vi "MTMount_putSample_AzimuthDrivesThermal.vi"(8 "error in (no error)":errorcluster, 11 "Azimuth_Drives_Thermal_Ctl":T1) -> (0 "error out":errorcluster, 2 "function return":i32, 3 "Azimuth_Drives_Thermal_Ctl out":T1)   [LabVIEW 2018, in "SALLV_MTMount.lvlib"]
doc: "int MTMount_shm_putSample_Azimuth_Drives_ThermalLV(MTMount_Azimuth_Drives_ThermalLV *Azimuth_Drives_Thermal_Ctl );"
uses:
  SALLV_MTMount.lvlib
  DataTypes/Azimuth_Drives_Thermal.ctl
  SALLV_MTMount.so
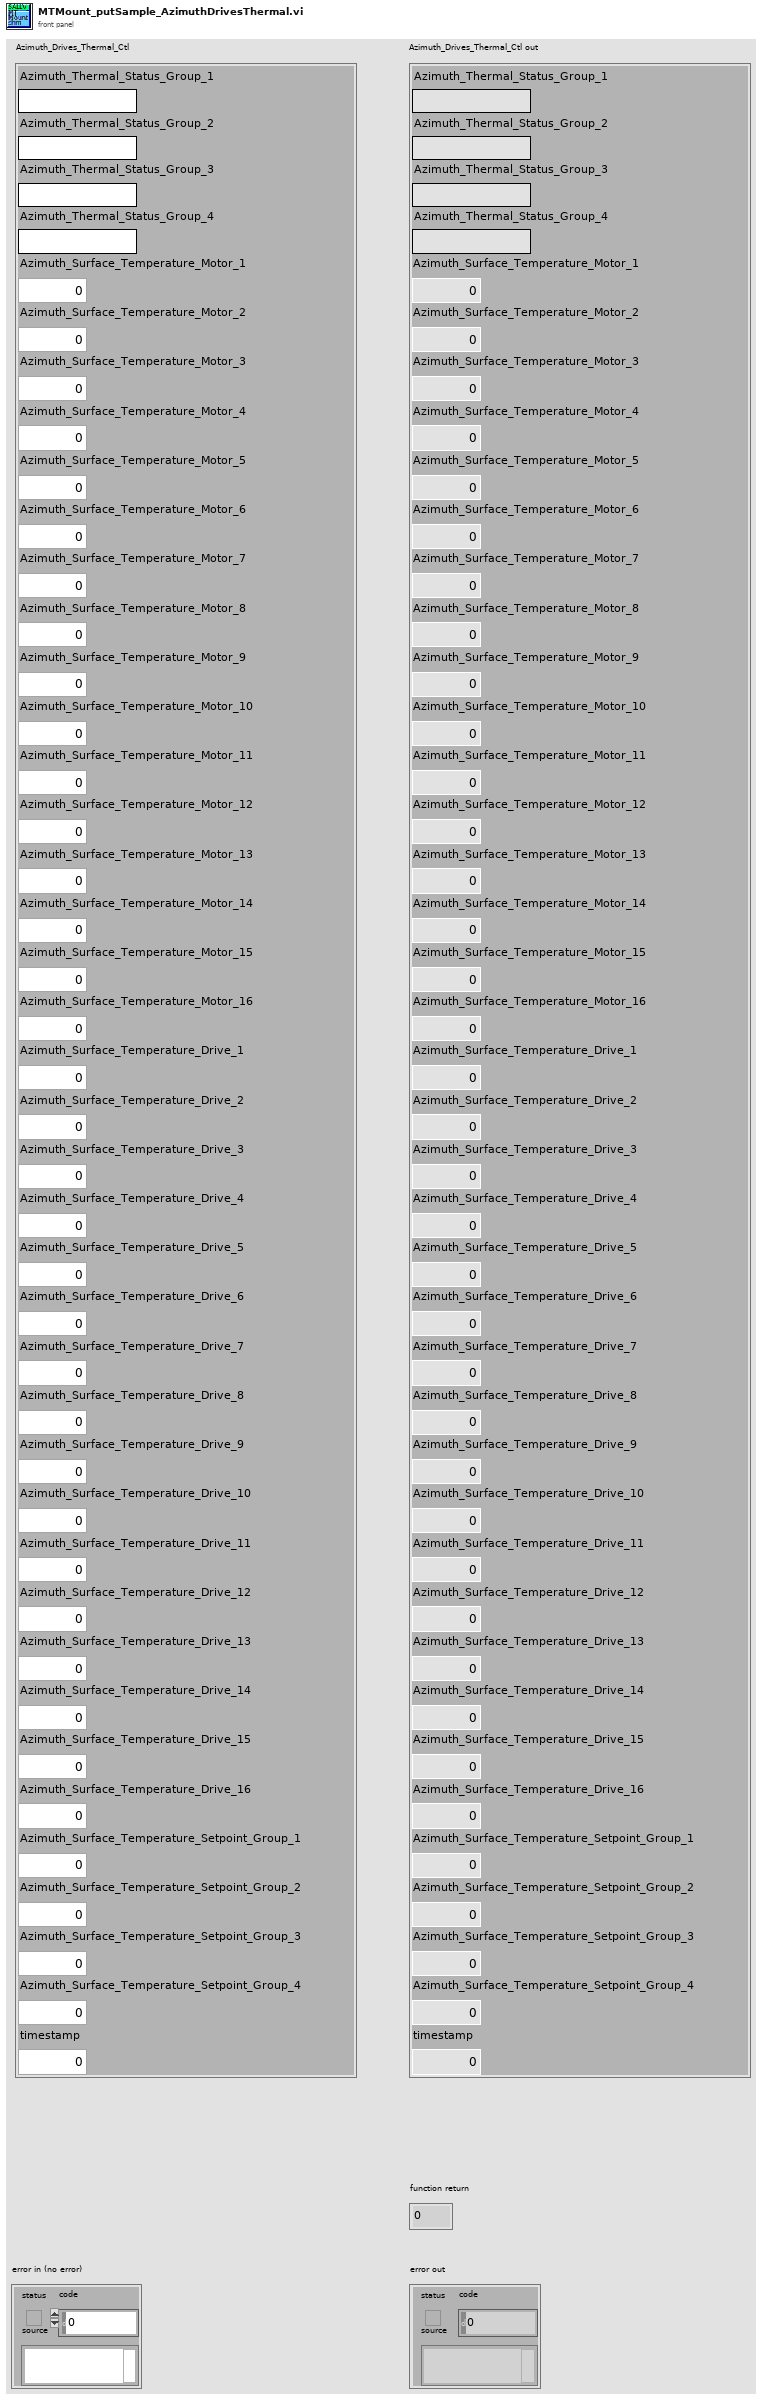
[diagram p1: front panel]
types:
  T1 = typedef "SALLV_MTMount.lvlib/Azimuth_Drives_Thermal.ctl" = cluster{"Azimuth_Thermal_Status_Group_1":string, "Azimuth_Thermal_Status_Group_2":string, "Azimuth_Thermal_Status_Group_3":string, "Azimuth_Thermal_Status_Group_4":string, "Azimuth_Surface_Temperature_Motor_1":dbl, "Azimuth_Surface_Temperature_Motor_2":dbl, "Azimuth_Surface_Temperature_Motor_3":dbl, "Azimuth_Surface_Temperature_Motor_4":dbl, "Azimuth_Surface_Temperature_Motor_5":dbl, "Azimuth_Surface_Temperature_Motor_6":dbl, "Azimuth_Surface_Temperature_Motor_7":dbl, "Azimuth_Surface_Temperature_Motor_8":dbl, "Azimuth_Surface_Temperature_Motor_9":dbl, "Azimuth_Surface_Temperature_Motor_10":dbl, "Azimuth_Surface_Temperature_Motor_11":dbl, "Azimuth_Surface_Temperature_Motor_12":dbl, "Azimuth_Surface_Temperature_Motor_13":dbl, "Azimuth_Surface_Temperature_Motor_14":dbl, "Azimuth_Surface_Temperature_Motor_15":dbl, "Azimuth_Surface_Temperature_Motor_16":dbl, "Azimuth_Surface_Temperature_Drive_1":dbl, "Azimuth_Surface_Temperature_Drive_2":dbl, "Azimuth_Surface_Temperature_Drive_3":dbl, "Azimuth_Surface_Temperature_Drive_4":dbl, "Azimuth_Surface_Temperature_Drive_5":dbl, "Azimuth_Surface_Temperature_Drive_6":dbl, "Azimuth_Surface_Temperature_Drive_7":dbl, "Azimuth_Surface_Temperature_Drive_8":dbl, "Azimuth_Surface_Temperature_Drive_9":dbl, "Azimuth_Surface_Temperature_Drive_10":dbl, "Azimuth_Surface_Temperature_Drive_11":dbl, "Azimuth_Surface_Temperature_Drive_12":dbl, "Azimuth_Surface_Temperature_Drive_13":dbl, "Azimuth_Surface_Temperature_Drive_14":dbl, "Azimuth_Surface_Temperature_Drive_15":dbl, "Azimuth_Surface_Temperature_Drive_16":dbl, "Azimuth_Surface_Temperature_Setpoint_Group_1":dbl, "Azimuth_Surface_Temperature_Setpoint_Group_2":dbl, "Azimuth_Surface_Temperature_Setpoint_Group_3":dbl, "Azimuth_Surface_Temperature_Setpoint_Group_4":dbl, "timestamp":dbl}
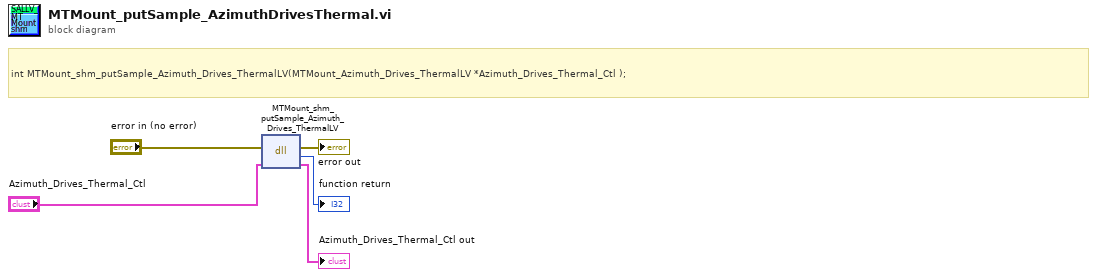
[diagram p0: block diagram]
diagram:
  # "int MTMount_shm_putSample_Azimuth_Drives_ThermalLV(MTMount_Azimuth_Drives_ThermalLV *Azimuth_Drives_Thermal_Ctl );"
  n1 = dll-call lib="home/ttsai/Document/salApiMTMount/SALLV_MTMount/SALLV_MTMount.*" fn="MTMount_shm_putSample_Azimuth_Drives_ThermalLV"(error in="error in (no error)", "Azimuth_Drives_Thermal_Ctl"="Azimuth_Drives_Thermal_Ctl") -> (error out=→"error out":errorcluster, →"function return":i32, "Azimuth_Drives_Thermal_Ctl"=→"Azimuth_Drives_Thermal_Ctl out":T1)  [unwired: 2 in, 1 out]
